vi "eval_free_pass.vi"(8 "error in (no error)":errorcluster, 11 "SN":string) -> (0 "error out":errorcluster, 2 "Device Type out":T1 items=["BGH Asset", "BGH Product", "SAMSUNG Product", "Generic Product", "No Product"], 3 "SN ok?":bool)   [LabVIEW 2024]
uses:
  controls/SN_device_type_out.ctl
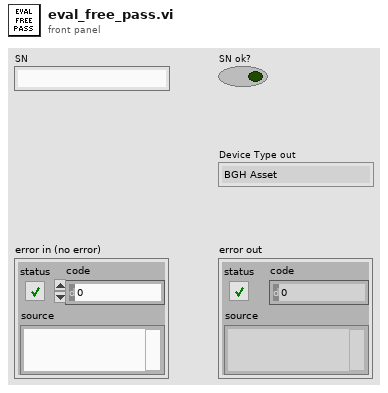
[diagram p1: front panel]
types:
  T1 = typedef "SN_device_type_out.ctl" = u16
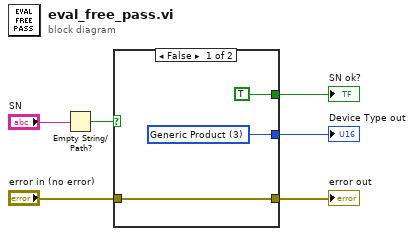
[diagram p0: block diagram]
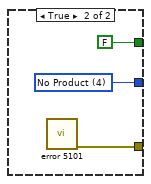
[diagram p2: hidden frame]
diagram:
  n1 = Empty String/Path?(string/path="SN") -> (empty?=w2:bool)
  n2 = case shown="False" w2 {
    tunnel: [w8 w11] -> w6
    tunnel: [TRUE FALSE] -> w5
    tunnel: [w7 w10] -> w3
    tunnel: "error in (no error)" -> [w7 _]
    frame False {
      w8 = T1 3 items=["BGH Asset", "BGH Product", "SAMSUNG Product", "Generic Product", "No Product"] ("Device Type out")
    }
    frame True {
      w11 = T1 4 items=["BGH Asset", "BGH Product", "SAMSUNG Product", "Generic Product", "No Product"] ("Device Type out")
      n3 = call "error 5101.vi"() -> ("error out"=w10:errorcluster)  [unwired: 11 in]
    }
  }
  "Device Type out" <- w6
  "SN ok?" <- w5
  "error out" <- w3
